vi "SaveConfig.vi"(11 "Config":T1={"Pico"="COM5", "Range"=enum."0.26", "Mode"=enum."Serial", "R"=[0.19948381185531616, 0.39327406883239746, 0.3932740092277527]}) -> ()   [LabVIEW 2025]
uses:
  Config.ctl
  Range.ctl
  Mode.ctl
  Globals.vi
panel:
  # "R1 Only"
  # "Parallel"
  # "Serial"
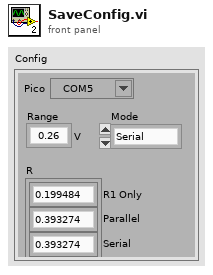
[diagram p1: front panel]
types:
  T1 = typedef "Config.ctl" = cluster{"Pico":refnum<visa-resource-name>, "Range":T2, "Mode":T3, "R":dbl[]}
  T2 = typedef "Range.ctl" = enum16{"0.26", "0.52", "1.03", "2.05", "4.1", "6.2"}
  T3 = typedef "Mode.ctl" = enum16{"R1 Only", "Parallel", "Serial"}
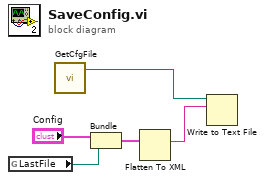
[diagram p0: block diagram]
diagram:
  n1 = global read "Globals.vi" "LastFile"() -> (w4:path)
  n2 = call "GetCfgFile.vi"() -> ("appended path"=w1:path)
  n3 = Bundle("Config"="Config", "LastFile"=w4) -> (w3:cluster{"Config":T1, "LastFile":path})  [unwired: 1 in]
  n4 = Flatten To XML(6:w3) -> (2:w2:string)
  n5 = Write to Text File(file (use dialog)=w1, text=w2) -> ()  [unwired: 2 in, 3 out]
